vi "AutoLowerArmTimeout.vi"(8 "error in (no error)":errorcluster, 10 "Timeout":u32=800, 11 "CollectorArmSpeed":dbl=1.0) -> (0 "error out":errorcluster, 3 "TimedOut?":bool)   [LabVIEW 2013]
uses:
  CollectorAction.ctl
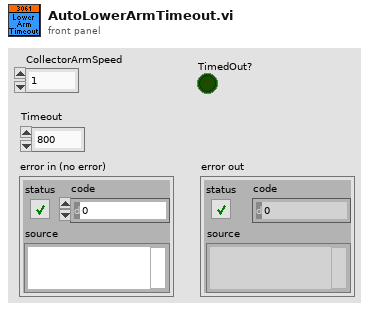
[diagram p1: front panel]
types:
  T1 = typedef "CollectorAction.ctl" = enum16{"Init", "Raise", "Lower", "Stop", "GetStatus"}
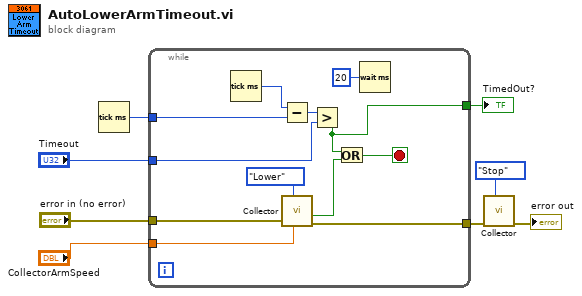
[diagram p0: block diagram]
diagram:
  n1 = Tick Count (ms)() -> (millisecond timer value=w7:u32)
  n2 = while {
    tunnel: "error in (no error)" -> [w9]
    tunnel: [w20] -> w3
    tunnel: w7 -> [w13]
    tunnel: "CollectorArmSpeed" -> [w12]
    tunnel: [w11] -> w4
    tunnel: "Timeout" -> [w10]
    stop <- w15 stop-if-true
    n3 = Tick Count (ms)() -> (millisecond timer value=w17:u32)
    n4 = Subtract(x=w17, y=w13) -> (x-y=w18:u32)
    n5 = call "Collector.vi"("MotorSpeed"=w12, "Action"=CollectorAction."Lower", "Error in"=w9) -> ("Error out"=w20:errorcluster, "Lower Triggered?"=w14:bool)  [unwired: 6 in, 1 out]
    n6 = Greater?(x=w18, y=w10) -> (0:w11:bool)
    n7 = Or(x=w11, y=w14) -> (x .or. y?=w15:bool)
    n8 = Wait (ms)(milliseconds to wait=u32 20) -> ()  [unwired: 1 out]
  }
  "TimedOut?" <- w4
  n9 = call "Collector.vi"("Action"=CollectorAction."Stop", "Error in"=w3) -> ("Error out"=→"error out":errorcluster)  [unwired: 7 in, 2 out]
